vi "CAL_FLOW_SENSOR 2016.vi"(7 "Array in":refnum<k24>[](array[refnum]), 8 "error in (no error)":errorcluster, 9 "Descriptions":string[](array[string]), 11 "flow_slope_IN":dbl=51.35 format="%.2f") -> (0 "error out":errorcluster, 2 "Sensor Cluster":T1, 3 "flow_slope\nmL/min":dbl=51.35 format="%.2f", 5 "Array out":refnum<k24>[](array[refnum]))   [LabVIEW 2016]
uses:
  C:/Program Files (x86)/National Instruments/LabVIEW 2016/vi.lib/ULx/ULx_LV.dll
  Waterloo DAQ/controls/MCC DAQ Readings.ctl
  KPRO_lv2015/ad interface/Global_SIM_switch.vi
  KPRO_lv2015/Kpro Globals.vi
panel:
  out "Flow":dbl format="%.2f"
  in  "stop":bool
  in  "start":bool
  # "FLOW SENSOR CALIBRATION"
  # "Start Kpro flow. Allow the flow to equilibrate."
  # "After flow has equilibrated,  Press Start, simultaneously move Kpro effluent into graduated cylinder."
  # "Press Stop when 100 mL of water has been collected."
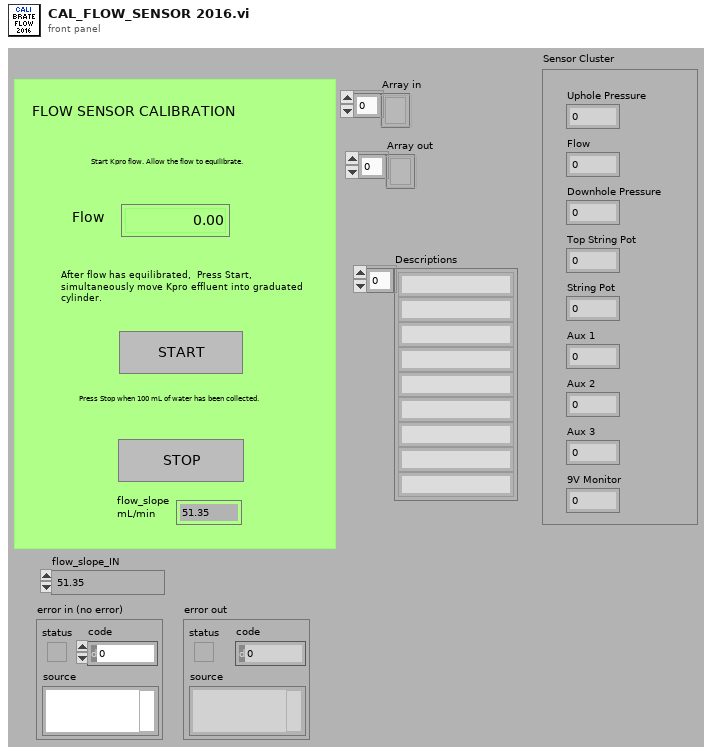
[diagram p1: front panel]
types:
  T1 = typedef "MCC DAQ Readings.ctl" = cluster{"Uphole Pressure":dbl, "Flow":dbl, "Downhole Pressure":dbl, "Top String Pot":dbl, "String Pot":dbl, "Aux 1":dbl, "Aux 2":dbl, "Aux 3":dbl, "9V Monitor":dbl}
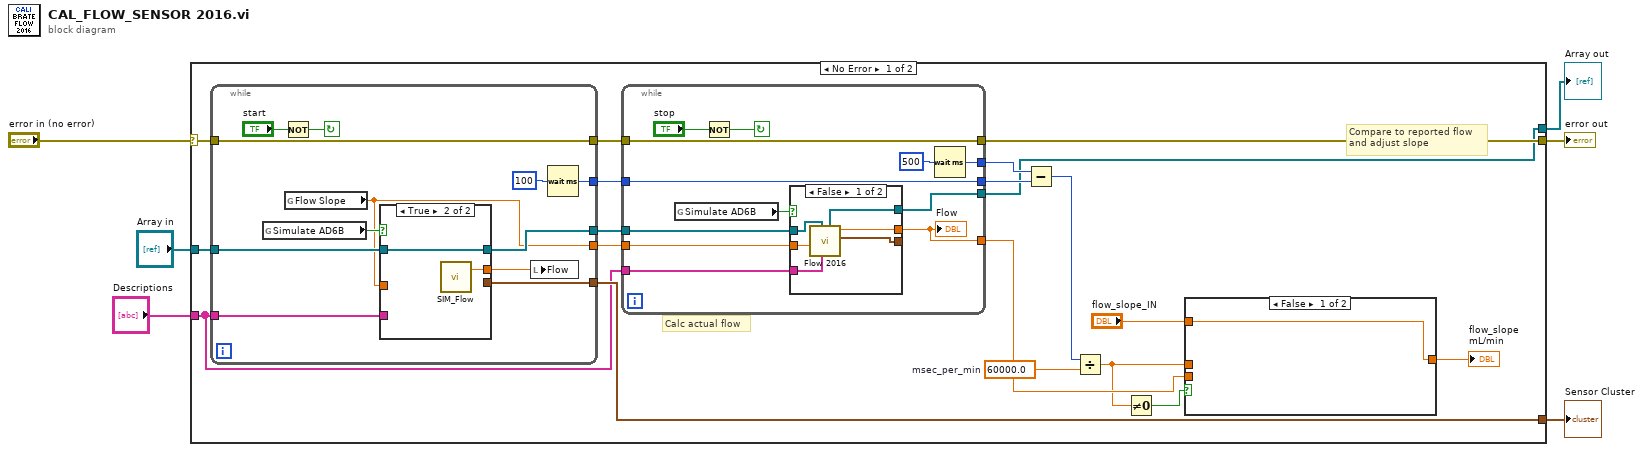
[diagram p0: block diagram]
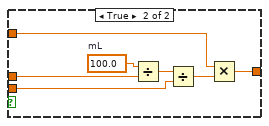
[diagram p2: hidden frame]
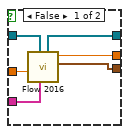
[diagram p3: hidden frame]
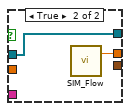
[diagram p4: hidden frame]
diagram:
  n1 = case shown="No Error" "error in (no error)" {
    selector: "error in (no error)" -> [w25 w75]
    tunnel: [w23 w75] -> w6
    tunnel: "Descriptions" -> [w12 _]
    tunnel: "Array in" -> [w14 w74]
    tunnel: [w13 _] -> w2
    tunnel: [w10 w74] -> w1
    frame No Error {
      w19 = 60000.0  # msec_per_min
      # "Compare to reported flow\nand adjust slope"
      # "Calc actual flow"
      n2 = while {
        tunnel: [w41] -> w24
        tunnel: w25 -> [w41]
        tunnel: [w42] -> w22
        tunnel: w12 -> [w38]
        tunnel: w14 -> [w37]
        tunnel: [w36] -> w13
        tunnel: [w35] -> w11
        tunnel: [w34] -> w9
        stop <- w44 continue-if-true
        n3 = global read "Global_SIM_switch.vi" "Simulate AD6B"() -> (w40:bool)
        n4 = Not(x="start") -> (.not. x?=w44:bool)
        n5 = global read "Kpro Globals.vi" "Flow Slope"() -> (w34:dbl)
        n6 = case shown="True" w40 {
          tunnel: [w48 w53] -> w39
          tunnel: w38 -> [w51 _]
          tunnel: w37 -> [w50 w52]
          tunnel: [w49 _] -> w36
          tunnel: w34 -> [w47 _]
          tunnel: [w46 w52] -> w35
          frame False {
            n7 = call "Flow 2016.vi"("Descriptions"=w51, "Array in"=w50, "Flow Slope"=w47) -> ("Sensor Cluster"=w49:T1, "Flow (ml/min)"=w48:dbl, "Array out"=w46:refnum<k24>[])  [unwired: 5 in]
          }
          frame True {
            n8 = call "SIM_Flow.vi"() -> ("Flow (ml/min)"=w53:dbl)  [unwired: 3 in]
          }
        }
        n9 = local write "Flow"(w39) -> ()
        n10 = Wait (ms)(milliseconds to wait=u32 100) -> (millisecond timer value=w42:u32)
      }
      n11 = while {
        tunnel: [w55] -> w15
        tunnel: w22 -> [w60]
        tunnel: [w60] -> w20
        tunnel: w24 -> [w61]
        tunnel: [w61] -> w23
        tunnel: [w63] -> w21
        tunnel: w12 -> [w58]
        tunnel: w11 -> [w57]
        tunnel: [w56] -> w10
        tunnel: w9 -> [w54]
        stop <- w65 continue-if-true
        n12 = global read "Global_SIM_switch.vi" "Simulate AD6B"() -> (w59:bool)
        n13 = Not(x="stop") -> (.not. x?=w65:bool)
        n14 = case shown="False" w59 {
          tunnel: [w68 w73] -> w55
          tunnel: w58 -> [w71 _]
          tunnel: w57 -> [w70 w72]
          tunnel: [w69 _] -> _
          tunnel: w54 -> [w67 _]
          tunnel: [w66 w72] -> w56
          frame False {
            n15 = call "Flow 2016.vi"("Descriptions"=w71, "Array in"=w70, "Flow Slope"=w67) -> ("Sensor Cluster"=w69:T1, "Flow (ml/min)"=w68:dbl, "Array out"=w66:refnum<k24>[])  [unwired: 5 in]
          }
          frame True {
            n16 = call "SIM_Flow.vi"() -> ("Flow (ml/min)"=w73:dbl)  [unwired: 3 in]
          }
        }
        "Flow" <- w55
        n17 = Wait (ms)(milliseconds to wait=u32 500) -> (millisecond timer value=w63:u32)
      }
      n18 = Subtract(x=w21, y=w20) -> (x-y=w18:u32)
      n19 = Divide(x=w18, y=w19) -> (x/y=w7:dbl)
      n20 = Not Equal To 0?(x=w7) -> (x != 0?=w8:bool)
      n21 = case shown="False" w8 {
        tunnel: w7 -> [_ w32]
        tunnel: "flow_slope_IN" -> [w26 w30]
        tunnel: [w26 w29] -> w16
        tunnel: w15 -> [_ w27]
        frame False {
        }
        frame True {
          w33 = 100.0  # mL
          n22 = Divide(x=w33, y=w32) -> (x/y=w28:dbl)
          n23 = Divide(x=w28, y=w27) -> (x/y=w31:dbl)
          n24 = Multiply(x=w30, y=w31) -> (x*y=w29:dbl)
        }
      }
      "flow_slope\nmL/min" <- w16
    }
    frame Error {
    }
  }
  "error out" <- w6
  "Sensor Cluster" <- w2
  "Array out" <- w1
